vi "Endpoint Aliases Page.vi"(8 "error in (no error)":errorcluster, 11 "Node Ptr":T5 format="%.0x") -> (0 "error out":errorcluster)   [LabVIEW 2020, in "Routing and Faulting System Explorer.lvlib"]
uses:
  Routing and Faulting System Explorer.lvlib
  <vilib>/NI VeriStand/Custom Device API/Custom Device Item Ref.ctl
  Alias.ctl
  Endpoint.ctl
  Shared/UI Common/Sort Button.ctl
  Shared/UI Common/Add Button.ctl
  Aliases Page Controls.ctl
  9b1be06d-3bcf-4b89-8ea1-6f7bb6167b61.vi
  Shared/UI Common/Set Control Value.vi
  <vilib>/NI VeriStand/Custom Device API/Custom Device API.lvlib
  Shared/UI Common/UI Common.lvlib
panel:
  in  "Items to add":dbl=5.0
  in  "Add Alias":T1
  in  "Sort":T2
  out "Alias":string="Alias"
  out "Endpoint":string="Endpoint"
  in  "Aliases":T3[](array[typedef])
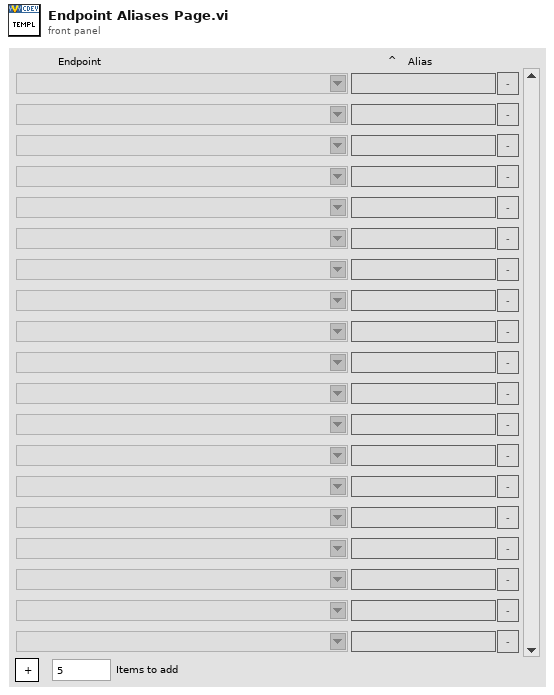
[diagram p1: front panel]
types:
  T1 = typedef "UI Common.lvlib/Add Button.ctl" = bool
  T2 = typedef "UI Common.lvlib/Sort Button.ctl" = bool
  T3 = typedef "Routing and Faulting System Explorer.lvlib/Alias.ctl" = cluster{"Endpoint":T4, "Alias":string, "Remove":bool}
  T4 = typedef "Routing and Faulting System Explorer.lvlib/Endpoint.ctl" = string
  T5 = typedef "Custom Device API.lvlib/Custom Device Item Ref.ctl" = u64
  T6 = typedef "Routing and Faulting System Explorer.lvlib/Aliases Page Controls.ctl" = cluster{"Aliases":refnum<vi>, "Endpoint":refnum<vi>, "Alias":refnum<vi>, "Sort":refnum<vi>}
  T7 = typedef "Custom Device API.lvlib/Custom Device Commands.ctl" = enum16{"Default", "Item renamed", "Shutdown", "Dynamic button pressed"}
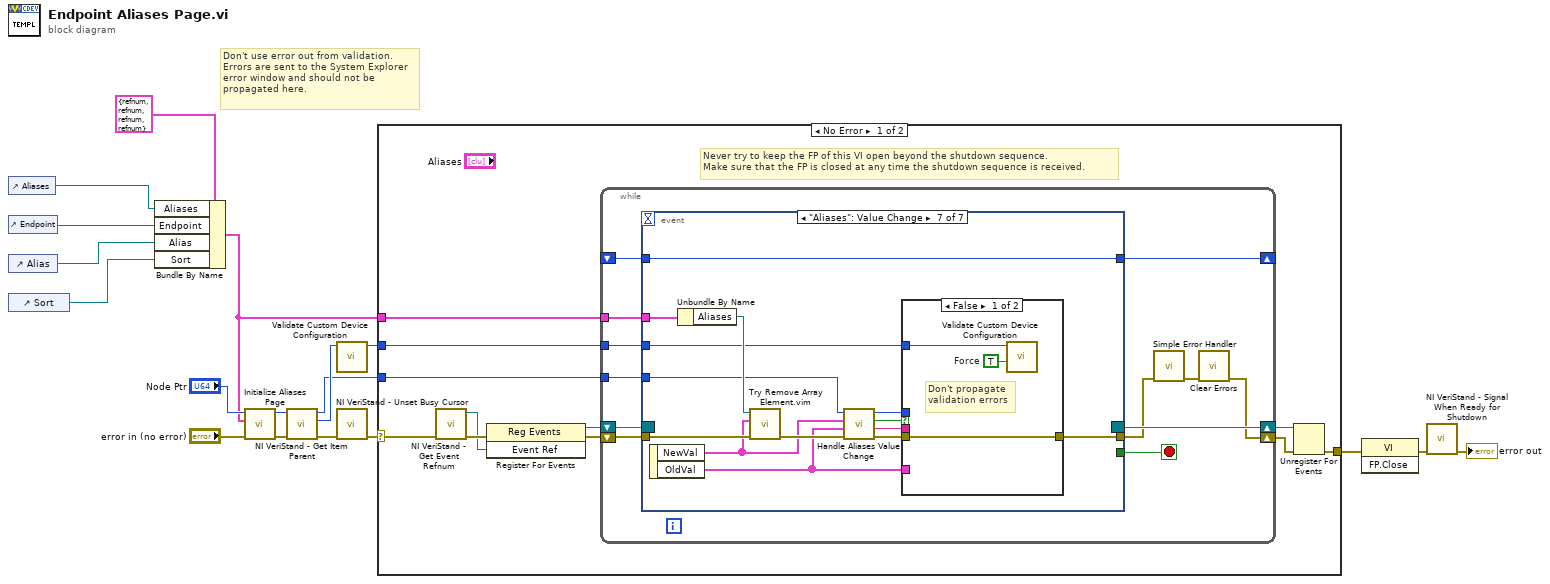
[diagram p0: block diagram]
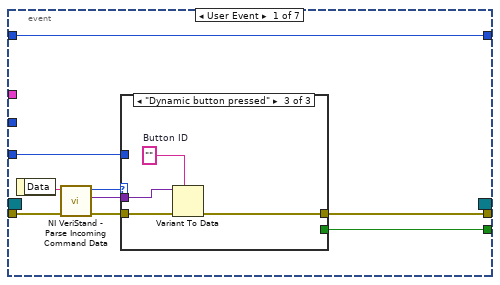
[diagram p2: hidden frame]
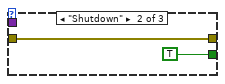
[diagram p4: hidden frame]
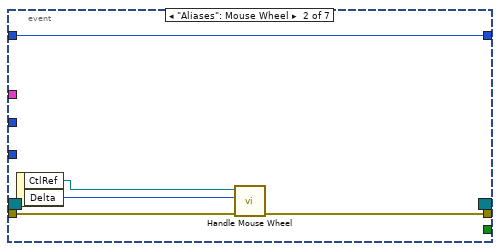
[diagram p5: hidden frame]
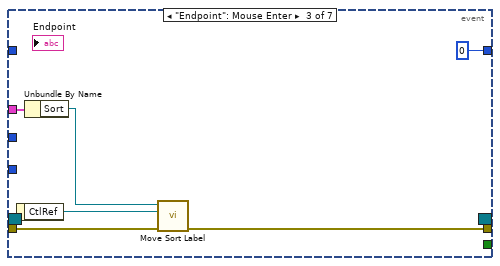
[diagram p6: hidden frame]
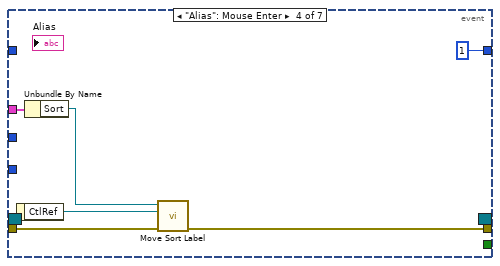
[diagram p7: hidden frame]
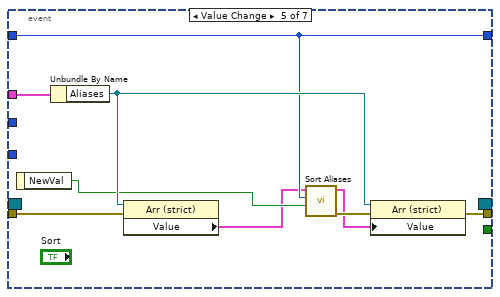
[diagram p8: hidden frame]
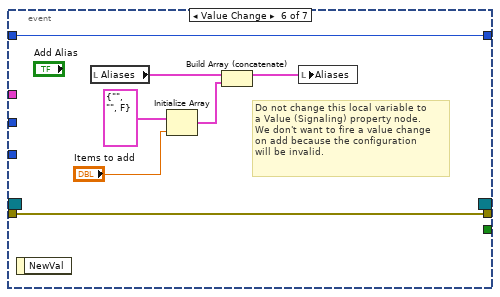
[diagram p9: hidden frame]
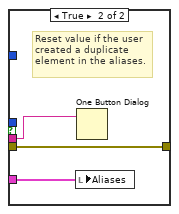
[diagram p10: hidden frame]
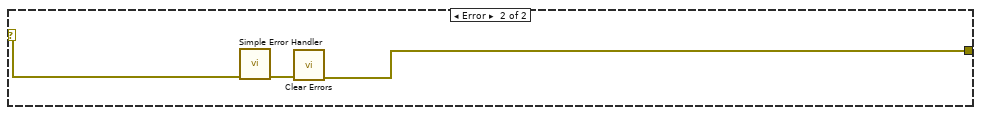
[diagram p11: hidden frame]
diagram:
  # "Don't use error out from validation.\nErrors are sent to the System Explorer\nerror window and should not be\npropagated here."
  n1 = control-ref of="Aliases"() -> (w7:refnum<vi>)
  n2 = control-ref of="Endpoint"() -> (w13:refnum<vi>)
  n3 = control-ref of="Alias"() -> (w12:refnum<vi>)
  n4 = control-ref of="Sort"() -> (w11:refnum<vi>)
  n5 = Bundle By Name(cluster=T6 {"Aliases"=refnum, "Endpoint"=refnum, "Alias"=refnum, "Sort"=refnum} ("Aliases Page Controls"), "Aliases"=w7, "Endpoint"=w13, "Alias"=w12, "Sort"=w11) -> (w8:T6)
  n6 = call "Initialize Aliases Page.vi"("error in (no error)"="error in (no error)", "Aliases Page Controls"=w8, "Aliases Ref in"="Node Ptr") -> ("error out"=w6:errorcluster, "Aliases Ref out"=w4:T5)  [unwired: 7 in]
  n7 = call <vilib>:"NI VeriStand - Get Item Parent.vi"("error in (no error)"=w6, "Item Ref in"=w4) -> ("error out"=w5:errorcluster, "Parent Ref"=w3:T5, "Item Ref out"=w2:T5)  [unwired: 6 in, 1 out]
  n8 = call "Validate Custom Device Configuration.vi"("Routing and Faulting Custom Device Ref"=w3) -> ("Routing and Faulting Custom Device Ref out"=w1:T5)  [unwired: 8 in, 2 out]
  n9 = call <vilib>:"NI VeriStand - Unset Busy Cursor.vi"("error in (no error)"=w5) -> ("error out"=w16:errorcluster)  [unwired: 10 out]
  n10 = case shown="No Error" w16 {
    selector: w16 -> [w25 w113]
    tunnel: [w27 w111] -> w18
    tunnel: w8 -> [w23 _]
    tunnel: w2 -> [w20 _]
    tunnel: w1 -> [w19 _]
    frame No Error {
      # "Never try to keep the FP of this VI open beyond the shutdown sequence.\nMake sure that the FP is closed at any time the shutdown sequence is received."
      n11 = call <vilib>:"NI VeriStand - Get Event Refnum.vi"("error in (no error)"=w25) -> ("error out"=w22:errorcluster, "Event Ref"=w21:refnum<user-event>)  [unwired: 9 out]
      n12 = register-events(error in=w22, w21) -> (reference out=w26:refnum<event-registration>, error out=w24:errorcluster)  [unwired: 1 in]
      n13 = while {
        shift-right: [w35] -> w28
        shift-left: w24 -> [w40]
        shift-right: [w41] -> w29
        shift-left: w26 -> [w39]
        shift-right: [w34] -> _
        shift-left: _ -> [w32]
        tunnel: w23 -> [w33]
        tunnel: w20 -> [w31]
        tunnel: w19 -> [w30]
        stop <- w38 stop-if-true
        n14 = event shown="[6] \"Aliases\": Value Change" {
          selector: w39 -> [_ _ _ _ _ _ _]
          dyn-events: [_ _ _ _ _ _ _] -> w41
          timeout: _ -> [_ _ _ _ _ _ _]
          tunnel: w40 -> [w50 w60 w68 w74 w83 w88 w103]
          tunnel: [w46 _ _ _ _ _ _] -> w38
          tunnel: [w45 w59 w67 w73 w80 w88 w93] -> w37
          tunnel: w31 -> [w44 _ _ _ _ _ w98]
          tunnel: [w42 w62 0 ("index of element") 1 ("index of element") w77 w90 w104] -> w34
          tunnel: w33 -> [_ _ w64 w70 w82 _ w102]
          tunnel: w32 -> [w42 w62 _ _ w77 w90 w104]
          tunnel: w30 -> [_ _ _ _ _ _ w91]
          event User Event {
            n15 = event-data() -> ("Data"=w49:string)  [unwired: 1 out]
            n16 = call <vilib>:"NI VeriStand - Parse Incoming Command Data.vi"("error in (no error)"=w50, "Incoming data"=w49) -> ("error out"=w48:errorcluster, "Outgoing data"=w43:variant, "Action"=w47:T7)  [unwired: 7 out]
            n17 = case shown="\"Dynamic button pressed\"" w47 {
              tunnel: w48 -> [w51 w52 w57]
              tunnel: [_ TRUE _] -> w46
              tunnel: [w51 w52 w54] -> w45
              tunnel: w44 -> [_ _ _]
              tunnel: w43 -> [_ _ w56]
              frame "Default", Default {
              }
              frame "Shutdown" {
              }
              frame "Dynamic button pressed" {
                w55 = ""  # Button ID
                n18 = Variant To Data(error in=w57, type=w55, Variant=w56) -> (error out=w54:errorcluster)  [unwired: 1 out]
              }
            }
          }
          event "Aliases": Mouse Wheel {
            n19 = event-data() -> ("CtlRef"=w61:refnum<vi>, "Delta"=w58:i32)  [unwired: 1 out]
            n20 = call "Handle Mouse Wheel.vi"("error in (no error)"=w60, "delta"=w58, "Array Refnum"=w61) -> ("error out"=w59:errorcluster)  [unwired: 7 in, 1 out]
          }
          event "Endpoint": Mouse Enter {
            n21 = event-data() -> ("CtlRef"=w66:refnum<vi>)  [unwired: 1 out]
            n22 = Unbundle By Name(w64) -> ("Sort"=w63:refnum<vi>)
            n23 = call "Move Sort Label.vi"("error in (no error)"=w68, "Target Label"=w66, "Sort"=w63) -> ("error out"=w67:errorcluster)  [unwired: 8 in]
          }
          event "Alias": Mouse Enter {
            n24 = event-data() -> ("CtlRef"=w72:refnum<vi>)  [unwired: 1 out]
            n25 = Unbundle By Name(w70) -> ("Sort"=w69:refnum<vi>)
            n26 = call "Move Sort Label.vi"("error in (no error)"=w74, "Target Label"=w72, "Sort"=w69) -> ("error out"=w73:errorcluster)  [unwired: 8 in]
          }
          event Value Change {
            n27 = event-data() -> ("NewVal"=w78:T2)  [unwired: 1 out]
            n28 = Unbundle By Name(w82) -> ("Aliases"=w79:refnum<vi>)
            n29 = property class="Arr (strict)"(reference=w79, error in=w83) -> ("Value"=w75:T3[])  [unwired: 2 out]
            n30 = call "Sort Aliases.vi"("Descending"=w78, "index"=w77, "Aliases"=w75) -> ("error out"=w81:errorcluster, "Sorted Aliases"=w76:T3[])  [unwired: 7 in]
            n31 = property class="Arr (strict)"(reference=w79, error in=w81, "Value"=w76) -> (error out=w80:errorcluster)  [unwired: 1 out]
          }
          event Value Change {
            # "Do not change this local variable to\na Value (Signaling) property node.\nWe don't want to fire a value change\non add because the configuration\nwill be invalid."
            n32 = event-data() -> ()  [unwired: 2 out]
            n33 = local read "Aliases"() -> (w86:T3[])
            n34 = Initialize Array(T3 {"Endpoint"="", "Alias"="", "Remove"=FALSE} ("Alias"), "Items to add") -> (w85:T3[])
            n35 = Build Array (concatenate)(w86, w85) -> (w84:T3[])
            n36 = local write "Aliases"(w84) -> ()
          }
          event "Aliases": Value Change {
            n37 = event-data() -> ("NewVal"=w99:T3[], "OldVal"=w96:T3[])  [unwired: 1 out]
            n38 = Unbundle By Name(w102) -> ("Aliases"=w101:refnum<vi>)
            n39 = call "Try Remove Array Element.vim"("error in (no error)"=w103, "Array"=w99, "Ctl Refnum"=w101) -> ("error out"=w100:errorcluster)  [unwired: 6 in, 2 out]
            n40 = call "Handle Aliases Value Change.vi"("error in (no error)"=w100, "OldVal"=w96, "NewVal"=w99, "Aliases Ref in"=w98) -> ("error out"=w97:errorcluster, "Duplicate Item"=w94:string, "Duplicate Entry"=w95:bool, "Aliases Ref out"=w92:T5)  [unwired: 4 in]
            n41 = case shown="False" w95 {
              tunnel: w97 -> [w105 w109]
              tunnel: w96 -> [_ w110]
              tunnel: [w105 w109] -> w93
              tunnel: w94 -> [_ w108]
              tunnel: w92 -> [_ _]
              tunnel: w91 -> [w107 _]
              frame False {
                w106 = TRUE  # Force
                # "Don't propagate\nvalidation errors"
                n42 = call "Validate Custom Device Configuration.vi"("Force Validation (F)"=w106, "Routing and Faulting Custom Device Ref"=w107) -> ()  [unwired: 7 in, 3 out]
              }
              frame True {
                # "Reset value if the user\ncreated a duplicate\nelement in the aliases."
                n43 = local write "Aliases"(w110) -> ()
                n44 = One Button Dialog(message=w108) -> ()  [unwired: 1 in, 1 out]
              }
            }
          }
        }
        n45 = call <vilib>:"Simple Error Handler.vi"("error in (no error)"=w37) -> ("error out"=w36:errorcluster)  [unwired: 1 in, 7 out]
        n46 = call <vilib>:"Clear Errors.vi"("error in (no error)"=w36) -> ("error out"=w35:errorcluster)  [unwired: 1 in, 5 out]
      }
      n47 = Unregister For Events(event registration refnum=w29, error in=w28) -> (error out=w27:errorcluster)
    }
    frame Error {
      n48 = call <vilib>:"Simple Error Handler.vi"("error in (no error)"=w113) -> ("error out"=w112:errorcluster)  [unwired: 1 in, 7 out]
      n49 = call <vilib>:"Clear Errors.vi"("error in (no error)"=w112) -> ("error out"=w111:errorcluster)  [unwired: 1 in, 5 out]
    }
  }
  n50 = invoke class="VI" method="FP.Close"(error in=w18) -> (error out=w10:errorcluster)  [unwired: 2 in, 2 out]
  n51 = call <vilib>:"NI VeriStand - Signal When Ready for Shutdown.vi"("error in (no error)"=w10) -> ("error out"=→"error out":errorcluster)  [unwired: 10 out]
